vi "FT_Get_Device_Serial_Number.vi"(0 "Handle":u32, 11 "Error In":errorcluster) -> (4 "FT_Status":u32(ring) items=["FT_OK", "FT_INVALID_HANDLE", "FT_DEVICE_NOT_FOUND", "FT_DEVICE_NOT_OPENED", "FT_IO_ERROR", "FT_INSUFFICIENT_RESOURCES", "FT_INVALID_PARAMETER", "FT_INVALID_BAUD_RATE", "FT_DEVICE_NOT_OPENED_FOR_ERASE", "FT_DEVICE_NOT_OPENED_FOR_WRITE", "FT_FAILED_TO_WRITE_DEVICE", "FT_EEPROM_READ_FAILED", "FT_EEPROM_WRITE_FAILED", "FT_EEPROM_ERASE_FAILED", "FT_EEPROM_NOT_PRESENT", "FT_EEPROM_NOT_PROGRAMMED", "FT_INVALID_ARGS", "FT_NOT_SUPPORTED", "FT_OTHER_ERROR"], 6 "SerialNumber":string, 15 "Error Out":errorcluster)   [LabVIEW 2016]
uses:
  FTD2XX.dll
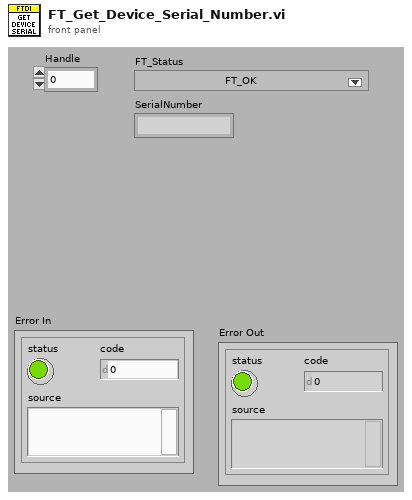
[diagram p1: front panel]
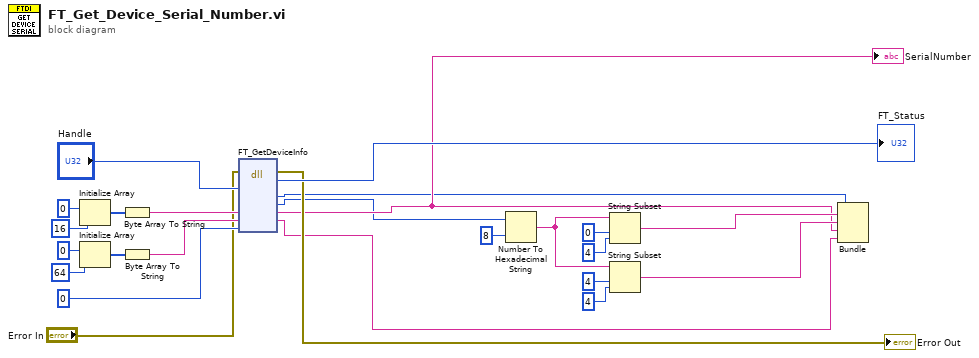
[diagram p0: block diagram]
diagram:
  n1 = Initialize Array(u8 0, 16 ("dimension size")) -> (w21:u8[])
  n2 = Initialize Array(u8 0, 64 ("dimension size")) -> (w19:u8[])
  n3 = Byte Array To String(unsigned byte array=w21) -> (string=w15:string)
  n4 = Byte Array To String(unsigned byte array=w19) -> (string=w16:string)
  n5 = dll-call lib="FTD2XX.dll" fn="FT_GetDeviceInfo"(error in="Error In", "Handle"="Handle", "SerialNumber"=w15, "Description"=w16, "Dummy"=u32 0) -> (error out=→"Error Out":errorcluster, "FT_Status"=→"FT_Status":u32, "DeviceType"=w1:u32, "ID"=w2:u32, "SerialNumber"=w3:string, "Description"=w4:string)  [unwired: 6 in, 1 out]
  "SerialNumber" <- w3
  n6 = Number To Hexadecimal String(1:i16 8 ("width (-)"), 2:w2) -> (0:w7:string)
  n7 = String Subset(string=w7, offset (0)=0, length (rest)=4 ("length (rest)")) -> (substring=w6:string)
  n8 = String Subset(string=w7, offset (0)=4, length (rest)=4 ("length (rest)")) -> (substring=w5:string)
  n9 = Bundle("DeviceType"=w1, w6, w5, "SerialNumber"=w3, "Description"=w4) -> ()  [unwired: 1 in, 1 out]
